vi "2D_Active_Target.vi"(6 "Iteration":i32, 8 "Active Plot":u32, 9 "Session":u32, 10 "XYGraph Refnum":refnum<vi>) -> (0 "y0":dbl, 1 "x0":dbl, 2 "Active Plot":u32, 3 "Radius":dbl)   [LabVIEW 2011]
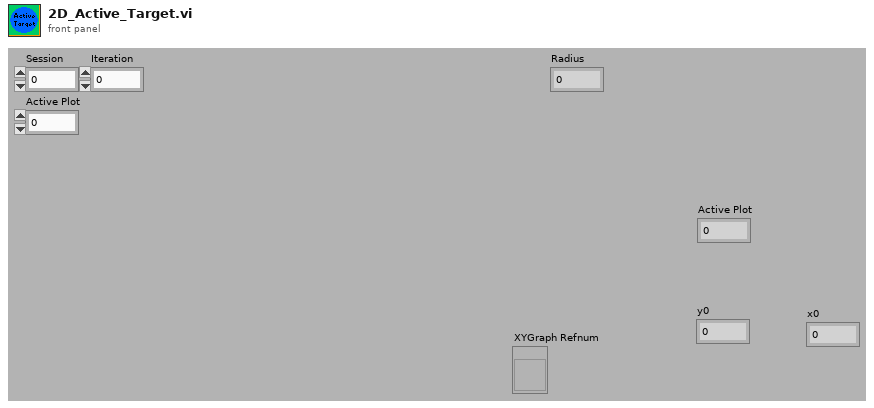
[diagram p1: front panel]
types:
  T1 = cluster{"Radius":dbl, "x0":dbl, "y0":dbl, "D":dbl, bool}
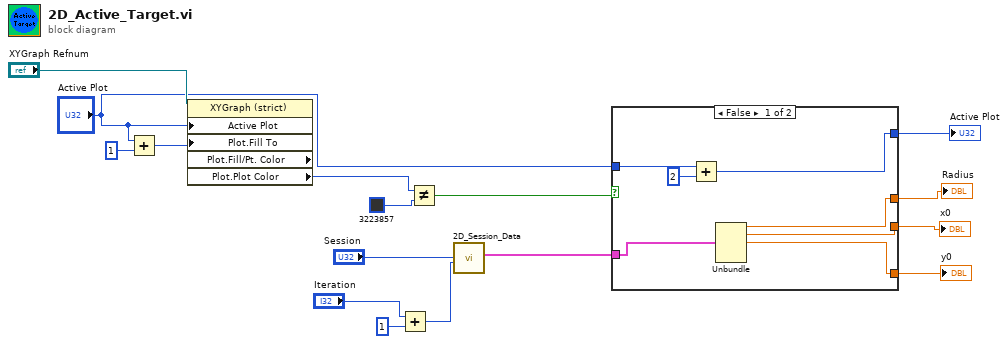
[diagram p0: block diagram]
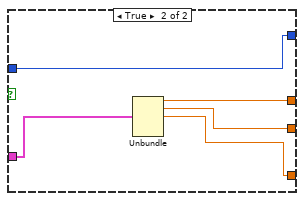
[diagram p2: hidden frame]
diagram:
  n1 = Add(x="Active Plot", y=u32 1) -> (x+y=w5:u32)
  n2 = property on="Property Node" class="XYGraph (strict)" props=["Active Plot", "Plot", "Fill To", "Plot", "Fill/Pt. Color", "Plot", "Plot Color"](reference="XYGraph Refnum", "Active Plot"="Active Plot", "Plot.Fill To"=w5) -> ("Plot.Plot Color"=w13:u32)  [unwired: 1 in, 3 out]
  n3 = Add(x="Iteration", y=1) -> (x+y=w1:i32)
  n4 = Not Equal?(x=w13, y=u32 3223857) -> (x != y?=w15:bool)
  n5 = call "2D_Session_Data.vi"("Iteration"=w1, "Session"="Session") -> ("output cluster"=w10:T1)  [unwired: 9 in]
  n6 = case shown="False" w15 {
    tunnel: [w20 w24] -> w16
    tunnel: w10 -> [w22 w28]
    tunnel: [w21 w27] -> w9
    tunnel: [w19 w26] -> w8
    tunnel: [w17 w25] -> w7
    tunnel: "Active Plot" -> [w18 w24]
    frame False {
      n7 = Add(x=w18, y=u32 2) -> (x+y=w20:u32)
      n8 = Unbundle(w22) -> ("Radius"=w21:dbl, "x0"=w19:dbl, "y0"=w17:dbl)  [unwired: 2 out]
    }
    frame True {
      n9 = Unbundle(w28) -> ("Radius"=w27:dbl, "x0"=w26:dbl, "y0"=w25:dbl)  [unwired: 2 out]
    }
  }
  "Active Plot" <- w16
  "x0" <- w8
  "y0" <- w7
  "Radius" <- w9
